vi "Get Run Rx Asynchronously.vi"(8 "error in":errorcluster, 11 "custom device":T1 format="%.0x") -> (0 "error out":errorcluster, 2 "run rx asynchronously":bool, 3 "custom device out":T1 format="%.0x")   [LabVIEW 2020, in "AIM MIL-STD-1553 Scripting.lvlib"]
doc: "Gets the state of the Run Rx Asynchronously boolean for the custom device."
uses:
  AIM MIL-STD-1553 Scripting.lvlib
  Constants.vi
  <vilib>/NI VeriStand/Custom Device API/Custom Device API.lvlib
  <vilib>/NI VeriStand/Custom Device API/Get Item Property (Boolean).vi
  <vilib>/NI VeriStand/Custom Device API/Custom Device Item Ref.ctl
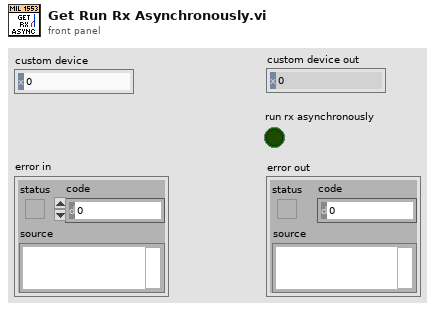
[diagram p1: front panel]
types:
  T1 = typedef "Custom Device API.lvlib/Custom Device Item Ref.ctl" = u64
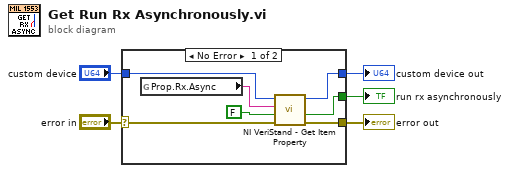
[diagram p0: block diagram]
diagram:
  n1 = case shown="No Error" "error in" {
    selector: "error in" -> [w9 w14]
    tunnel: [w8 w14] -> w2
    tunnel: [w11 w13] -> w3
    tunnel: "custom device" -> [w12 w13]
    tunnel: [w7 _] -> w5
    frame No Error {
      n2 = global read "Constants.vi" "Prop.Rx.Async"() -> (w10:string)
      n3 = call-poly <vilib>:"NI VeriStand - Get Item Property.vi"("error in (no error)"=w9, "Default Value"=FALSE, "Property Name"=w10, "Item Ref in"=w12) -> ("error out"=w8:errorcluster, "Value"=w7:bool, "Item Ref out"=w11:T1)  [unwired: 4 in, 1 out]
    }
    frame Error {
    }
  }
  "custom device out" <- w3
  "error out" <- w2
  "run rx asynchronously" <- w5
